vi "Write Part ID.vi"(8 "error in (no error)":errorcluster, 10 "Part ID":string, 11 "Thermistor1 in":refnum<class "Thermistor1.lvclass">) -> (0 "error out":errorcluster, 3 "Thermistor1 out":refnum<class "Thermistor1.lvclass">)   [LabVIEW 2024, in "Thermistor1.lvclass"]
uses:
  Thermistor1.lvclass
  Thermistor1.lvclass/Thermistor1.ctl
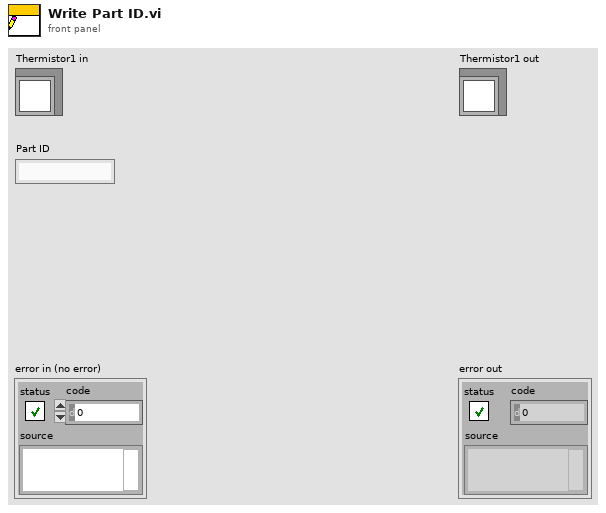
[diagram p1: front panel]
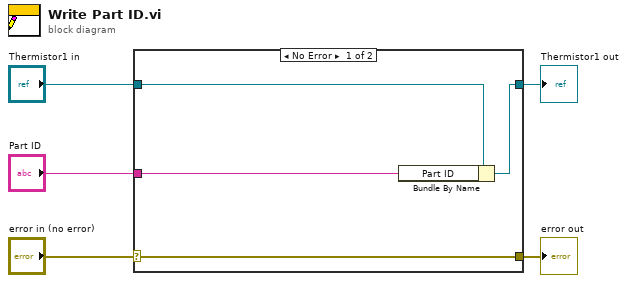
[diagram p0: block diagram]
diagram:
  n1 = case shown="No Error" "error in (no error)" {
    selector: "error in (no error)" -> [w9 w10]
    tunnel: [w9 w10] -> w4
    tunnel: [w7 w11] -> w2
    tunnel: "Thermistor1 in" -> [w8 w11]
    tunnel: "Part ID" -> [w6 _]
    frame No Error {
      n2 = Bundle By Name(cluster=w8, "Part ID"=w6) -> (w7:refnum<class "Thermistor1.lvclass">)
    }
    frame Error {
    }
  }
  "error out" <- w4
  "Thermistor1 out" <- w2
